vi "Disable Engine Run.vi"(6 "error in":errorcluster, 8 "MaxRead":i32, 9 "Channel in":u16) -> (0 "error out":errorcluster, 1 "Messages":T1(array[cluster]), 2 "Pass":bool, 3 "Channel out":u16)   [LabVIEW 2023]
uses:
  1c7e7734-3c4d-4630-804a-ed24e9547189.vi
  Communication/PCAN2023/PCAN API.lvlib
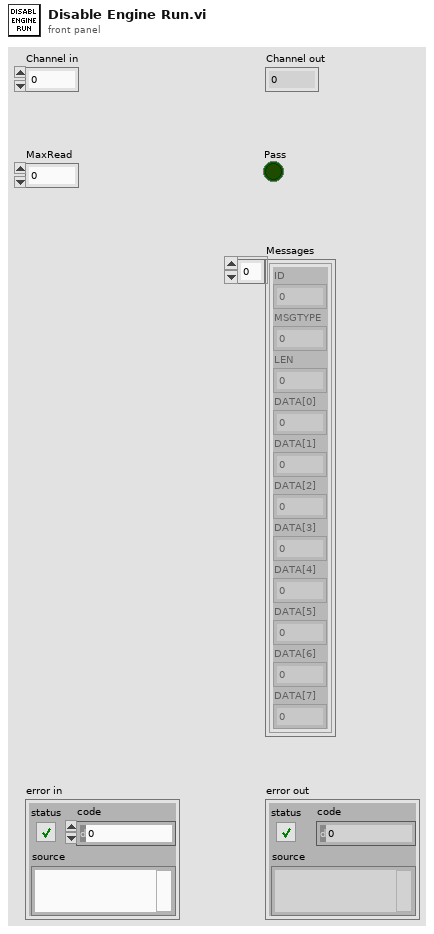
[diagram p1: front panel]
types:
  T1 = cluster{"ID":u32, "MSGTYPE":u8, "LEN":u8, "DATA[0]":u8, "DATA[1]":u8, "DATA[2]":u8, "DATA[3]":u8, "DATA[4]":u8, "DATA[5]":u8, "DATA[6]":u8, "DATA[7]":u8}[]
  T2 = cluster{"ID":u32, "MSGTYPE":u8, "LEN":u8, "DATA[0]":u8, "DATA[1]":u8, "DATA[2]":u8, "DATA[3]":u8, "DATA[4]":u8, "DATA[5]":u8, "DATA[6]":u8, "DATA[7]":u8}
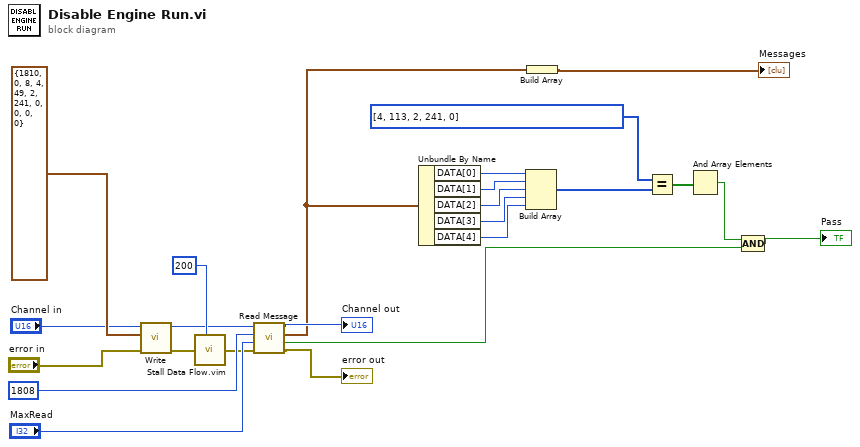
[diagram p0: block diagram]
diagram:
  n1 = call "Write.vi"("error in"="error in", "MessageBuffer"=T2 {"ID"=1810, "MSGTYPE"=0, "LEN"=8, "DATA[0]"=4, "DATA[1]"=49, "DATA[2]"=2, "DATA[3]"=241, "DATA[4]"=0, "DATA[5]"=0, "DATA[6]"=0, "DATA[7]"=0}, "Channel"="Channel in") -> ("error out"=w23:errorcluster, "Channel out"=w8:u16)  [unwired: 5 in, 2 out]
  n2 = call "Stall Data Flow.vim"("value in"=w23, "milliseconds to wait"=u32 200) -> ("value out"=w1:errorcluster)  [unwired: 1 out]
  n3 = call "Read Message.vi"("error in"=w1, "MaxRead"="MaxRead", "ID"=u32 1808, "Channel in"=w8) -> ("error out"=→"error out":errorcluster, "Passed"=w5:bool, "Last Message"=w4:T2, "Channel out"=→"Channel out":u16)  [unwired: 3 in, 1 out]
  n4 = Unbundle By Name(w4) -> ("DATA[0]"=w18:u8, "DATA[1]"=w17:u8, "DATA[2]"=w16:u8, "DATA[3]"=w15:u8, "DATA[4]"=w14:u8)
  n5 = Build Array(w18, w17, w16, w15, w14) -> (w12:u8[])
  n6 = Build Array(w4) -> (→"Messages":T1)
  n7 = Equal?(x=u8[] [4, 113, 2, 241, 0], y=w12) -> (x = y?=w11:bool[])
  n8 = And Array Elements(Boolean array=w11) -> (logical AND=w10:bool)
  n9 = Compound Arithmetic op=AND(w10, w5) -> (→"Pass":bool)
